vi "Velocity Get.vi"(8 "error in (no error)":errorcluster) -> (0 "error out":errorcluster, 2 "Velocity":T1 {"vz (mm/s)" format="%.1f"; "vy (mm/s)" format="%.1f"; "vx (mm/s)" format="%.1f"})   [LabVIEW 2019, in "Haptic Prog Interface.lvlib"]
doc: "Returns the velocities of the haptic pen in mm/s, and isn't dependent on the frame size.\n\n<b>Velocity:</b> Returns a cluster of the x, y, and z velocities of the pen (in units of mm/ss)."
uses:
  Haptic Prog Interface.lvlib
  src/x64/Debug/Haptic Programming Interface.dll
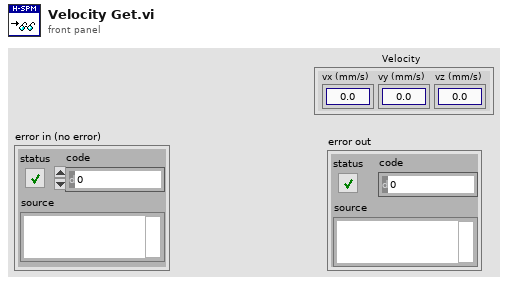
[diagram p1: front panel]
types:
  T1 = cluster{"vx (mm/s)":dbl, "vy (mm/s)":dbl, "vz (mm/s)":dbl}
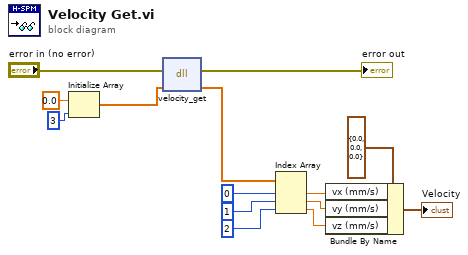
[diagram p0: block diagram]
diagram:
  n1 = Initialize Array(0.0 ("element"), 3 ("dimension size")) -> (w1:dbl[])
  n2 = dll-call lib="C:/Users/freem/Documents/GitHub/HapticSPM/Haptic-Programming-Interface/src/x64/Debug/Haptic Programming Interface.dll" fn="velocity_get"(error in="error in (no error)", "output"=w1) -> (error out=→"error out":errorcluster, "output"=w12:dbl[])  [unwired: 3 in, 1 out]
  n3 = Index Array(array=w12, index #1=0 ("index"), index #2=1 ("index"), index #3=2 ("index")) -> (element #1=w8:dbl, element #2=w7:dbl, element #3=w6:dbl)
  n4 = Bundle By Name(cluster=T1 {"vx (mm/s)"=0.0, "vy (mm/s)"=0.0, "vz (mm/s)"=0.0} ("Velocity"), "vx (mm/s)"=w8, "vy (mm/s)"=w7, "vz (mm/s)"=w6) -> (→"Velocity":T1)
